vi "ConvertExpressionDigits.vi"(11 "input":string) -> (3 "output":string)   [LabVIEW 2017, in "Trigger.lvlib"]
uses:
  <vilib>/addons/InsightCM/Devices/Shared/Common/Trigger/Trigger.lvlib
  <vilib>/regexp/Match Regular Expression.xnode
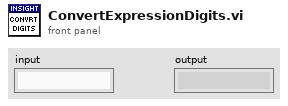
[diagram p1: front panel]
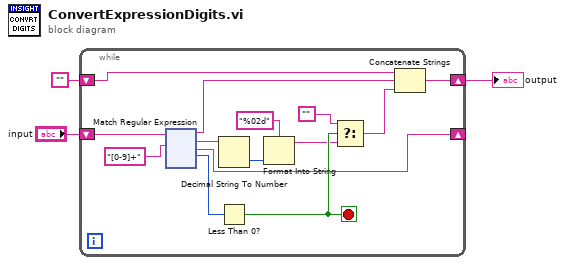
[diagram p0: block diagram]
diagram:
  n1 = while {
    shift-right: [w4] -> _
    shift-left: "input" -> [w16]
    shift-right: [w14] -> w1
    shift-left: "" -> [w15]
    stop <- w8 stop-if-true
    n2 = xnode "Match Regular Expression"("input string"=w16, "regular expression"="[0-9]+") -> ("before match"=w9:string, "whole match"=w10:string, "after match"=w4:string, "offset past match"=w17:i32)  [unwired: 4 in, 1 out]
    n3 = Decimal String To Number(string=w10) -> (number=w13:i32)  [unwired: 2 in, 1 out]
    n4 = Less Than 0?(x=w17) -> (x < 0?=w8:bool)
    n5 = Format Into String(format string="%02d", w13) -> (resulting string=w6:string)  [unwired: 2 in, 1 out]
    n6 = Select(t="", s=w8, f=w6) -> (s? t:f=w5:string)
    n7 = Concatenate Strings(w15, w9, w5) -> (w14:string)
  }
  "output" <- w1
